vi "selectable tc alarm.vi"(4 "Red Limit":dbl, 5 "Linearized Temperature":sgl, 6 "T ref":bool, 7 "Array Out Main in":dbl[](array[numeric]), 8 "Tc Alarm":bool, 9 "Target":dbl format="%0.2f", 10 "Yellow Limit":dbl, 11 "Numeric":dbl) -> (0 "Alarm Output":bool[](array[boolean]), 1 "Tref":dbl format="%#_13g", 2 "MA":dbl format="%#_13g", 3 "Array Out Main out":dbl[](array[numeric]))   [LabVIEW 2014]
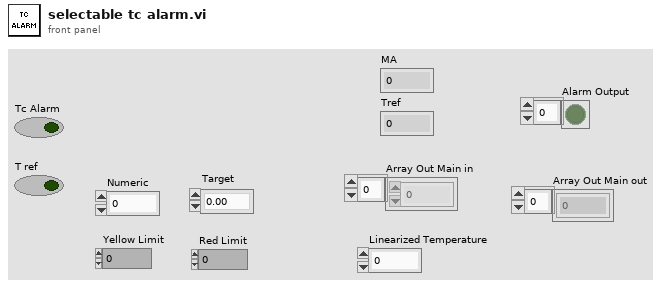
[diagram p1: front panel]
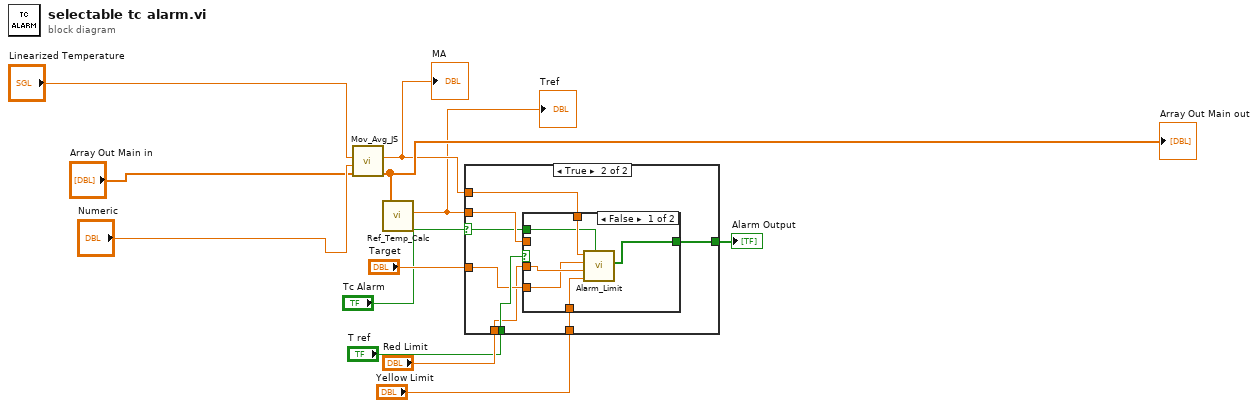
[diagram p0: block diagram]
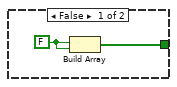
[diagram p2: hidden frame]
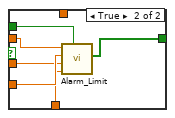
[diagram p3: hidden frame]
diagram:
  n1 = call "Mov_Avg_JS.vi"("Array In"="Array Out Main in", "Cycle Length"="Numeric", "Input"="Linearized Temperature") -> ("Array Out Main"=w7:dbl[], "Mean"=w2:dbl)  [unwired: 7 in]
  "Array Out Main out" <- w7
  "MA" <- w2
  n2 = call "Ref_Temp_Calc.vi"("Temp Array"=w7) -> ("T Ref"=w1:dbl)  [unwired: 10 in]
  "Tref" <- w1
  n3 = case shown="True" "Tc Alarm" {
    selector: "Tc Alarm" -> [_ w17]
    tunnel: "T ref" -> [_ w22]
    tunnel: [w13 w16] -> w3
    tunnel: w1 -> [_ w21]
    tunnel: "Target" -> [_ w20]
    tunnel: "Yellow Limit" -> [_ w19]
    tunnel: "Red Limit" -> [_ w18]
    tunnel: w2 -> [_ w15]
    frame False {
      w14 = FALSE
      n4 = Build Array(w14, w14) -> (w13:bool[])
    }
    frame True {
      n5 = case shown="False" w22 {
        tunnel: w21 -> [_ w34]
        tunnel: w20 -> [w26 w33]
        tunnel: w19 -> [w28 w32]
        tunnel: w18 -> [w27 w31]
        tunnel: w17 -> [w24 w30]
        tunnel: [w23 w29] -> w16
        tunnel: w15 -> [w25 _]
        frame False {
          n6 = call "Alarm_Limit.vi"("Alarm On"=w24, "Yellow Limit"=w28, "Red Limit"=w27, "Target"=w26, "Reading"=w25) -> ("Alarm Output"=w23:bool[])  [unwired: 6 in]
        }
        frame True {
          n7 = call "Alarm_Limit.vi"("Alarm On"=w30, "Yellow Limit"=w32, "Red Limit"=w31, "Target"=w33, "Reading"=w34) -> ("Alarm Output"=w29:bool[])  [unwired: 6 in]
        }
      }
    }
  }
  "Alarm Output" <- w3
